vi "avToStateImageAv.vi"(1 "attribute value":T1={"device name"="", "attribute name"="", "quality value"=0, "quality string"="", "timestamp"=0.0, "dim. x"=0, "dim. y"=0, "value"=[], "error code"=0, "error stack"=[], "data type"=36}) -> (0 "av":T2={"device name"="", "attribute name"="", "quality value"=0, "quality string"="", "timestamp"=0.0, "dim. x"=0, "dim. y"=0, "value"=[], "error code"=0, "error stack"=[], "data type"=36})   [LabVIEW 2014, in "tango.lvlib"]
uses:
  tango.lvlib
  base/toStateImage.vi
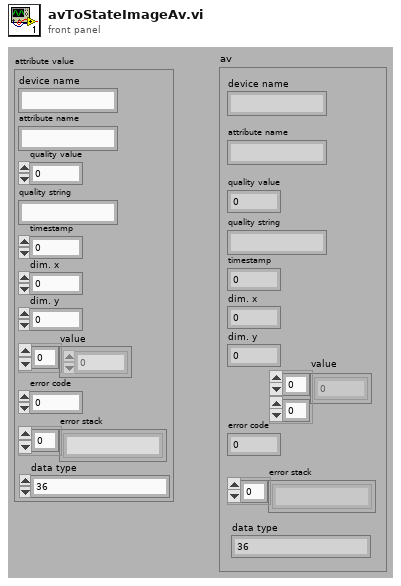
[diagram p1: front panel]
types:
  T1 = cluster{"device name":string, "attribute name":string, "quality value":i16, "quality string":string, "timestamp":dbl, "dim. x":i32, "dim. y":i32, "value":u8[], "error code":i32, "error stack":string[], "data type":u16}
  T2 = cluster{"device name":string, "attribute name":string, "quality value":i16, "quality string":string, "timestamp":dbl, "dim. x":i32, "dim. y":i32, "value":u8[][], "error code":i32, "error stack":string[], "data type":u16}
  T3 = typedef "tango.lvlib/_TangoState_t.ctl" = enum32{"ON", "OFF", "CLOSE", "OPEN", "INSERT", "EXTRACT", "MOVING", "STANDBY", "FAULT", "INIT", "RUNNING", "ALARM", "DISABLE", "UNKNOWN"}
  T4 = cluster{"device name":string, "attribute name":string, "quality value":i16, "quality string":string, "timestamp":dbl, "dim. x":i32, "dim. y":i32, "value_out":T3[][], "error code":i32, "error stack":string[], "data type":u16}
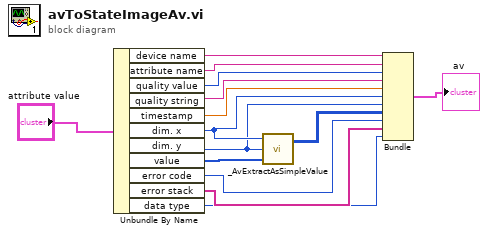
[diagram p0: block diagram]
diagram:
  n1 = Unbundle By Name("attribute value") -> ("device name"=w13:string, "attribute name"=w12:string, "quality value"=w11:i16, "quality string"=w10:string, "timestamp"=w9:dbl, "dim. x"=w3:i32, "dim. y"=w2:i32, "value"=w14:u8[], "error code"=w7:i32, "error stack"=w6:string[], "data type"=w1:u16)
  n2 = call-poly "_AvExtractAsSimpleValue.vi"("value_in"=w14, "dim_y"=w2, "dim_x"=w3) -> ("value_out"=w8:T3[][])  [unwired: 1 out]
  n3 = Bundle("device name"=w13, "attribute name"=w12, "quality value"=w11, "quality string"=w10, "timestamp"=w9, "dim. x"=w3, "dim. y"=w2, "value_out"=w8, "error code"=w7, "error stack"=w6, "data type"=w1) -> (→"av":T4)  [unwired: 1 in]
